vi "Start.vi"(8 "error in (no error)":errorcluster, 10 "Message in":refnum<class "StartMessage.lvclass">, 11 "RSA in":refnum<class "RSA.lvclass">) -> (0 "error out":errorcluster, 3 "RSA out":refnum<class "RSA.lvclass">)   [LabVIEW 2012, in "RSA.lvclass"]
doc: "This member function is called when the statemachine in the run.vi receives an 'start' command. It relays the message to all observers of the component.\n\nOverride this member function in your derived class if you need additional start functionality (but don't forget to call the parent method)."
uses:
  RSA.lvclass
  <vilib>/Distrio/Murmex/StartMessage/StartMessage.lvclass
  <vilib>/Distrio/Murmex/Murmex/Murmex.lvclass
  <vilib>/Distrio/Murmex/ProceedMessage/ProceedMessage.lvclass
  RSA.lvclass/RSA.ctl
panel:
  # "This member function is called when the statemachine in the run.vi receives an 'start' command. It relays the message to all observers of the component.\n\nOverride this member function in your derived class if you need additional start functionality (but don't forget to call the parent method)."
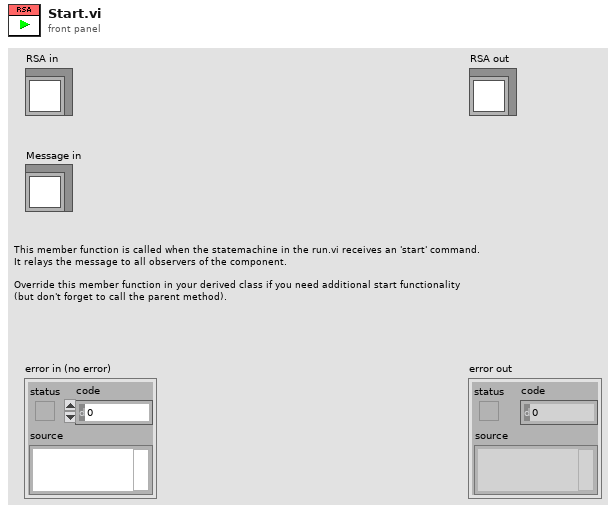
[diagram p1: front panel]
types:
  T1 = typedef "RSA.lvclass/starting shape.ctl" = enum16{"Load shape", "Midrange"}
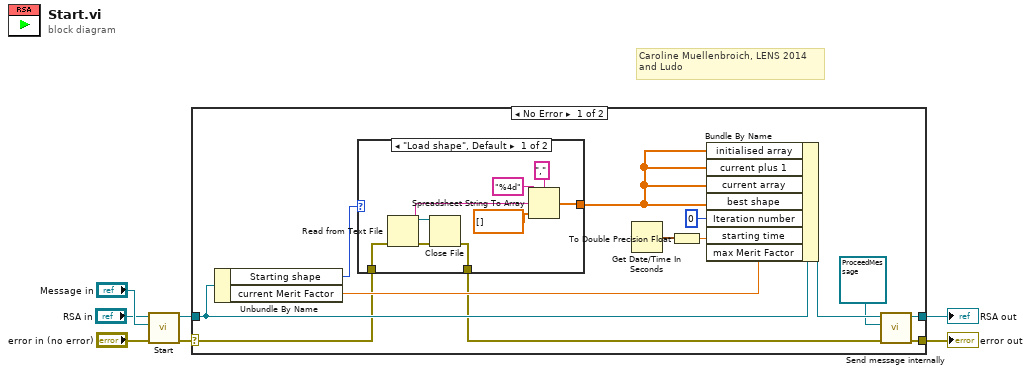
[diagram p0: block diagram]
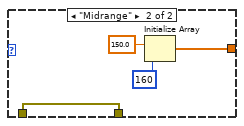
[diagram p2: hidden frame]
diagram:
  # "Caroline Muellenbroich, LENS 2014\nand Ludo"
  n1 = call-parent "Start.vi"("error in (no error)"="error in (no error)", "Message in"="Message in", "Murmex in"="RSA in") -> ("error out"=w4:errorcluster, "Murmex out"=w3:refnum<class "RSA.lvclass">)  [unwired: 7 in]
  n2 = case shown="No Error" w4 {
    selector: w4 -> [w9 w34]
    tunnel: w3 -> [w20 w35]
    tunnel: [w16 w35] -> w2
    tunnel: [w17 w34] -> w1
    frame No Error {
      n3 = Unbundle By Name(w20) -> ("Starting shape"=w11:T1, "current Merit Factor"=w12:dbl)
      n4 = case shown="\"Load shape\", Default" w11 {
        tunnel: [w24 w31] -> w10
        tunnel: w9 -> [w23 w30]
        tunnel: [w21 w30] -> w8
        frame "Load shape", Default {
          n5 = Read from Text File(error in=w23) -> (refnum out=w26:refnum<file>, text=w29:string, error out=w22:errorcluster)  [unwired: 1 in, 3 out]
          n6 = Close File(refnum=w26, error in=w22) -> (error out=w21:errorcluster)  [unwired: 1 out]
          n7 = Spreadsheet String To Array(delimiter (Tab)=",", format string="%4d", spreadsheet string=w29, array type (2D Dbl)=dbl[] [] ("run time Cluster.1x160  Voltage Map")) -> (array=w24:dbl[])
        }
        frame "Midrange" {
          n8 = Initialize Array(150.0 ("element"), 160 ("dimension size")) -> (w31:dbl[])
        }
      }
      n9 = Get Date/Time In Seconds() -> (seconds since 1Jan1904=w19:timestamp)
      n10 = To Double Precision Float(number=w19) -> (double precision float=w18:dbl)
      n11 = Bundle By Name(cluster=w20, "initialised array"=w10, "current plus 1"=w10, "current array"=w10, "best shape"=w10, "Iteration number"=0 ("Run time cluster.Iteration number"), "starting time"=w18, "max Merit Factor"=w12) -> (w15:refnum<class "RSA.lvclass">)
      n12 = call <vilib>:"Send message internally.vi"("error in (no error)"=w8, "Message"=refnum<class "ProceedMessage.lvclass"> refnum ("ProceedMessage"), "Murmex in"=w15) -> ("error out"=w17:errorcluster, "Murmex out"=w16:refnum<class "RSA.lvclass">)  [unwired: 7 in]
    }
    frame Error {
    }
  }
  "error out" <- w1
  "RSA out" <- w2
